vi "parseFloatFromLine.vi"(8 "error in (no error)":errorcluster, 9 "engineeringStatus":string, 10 "line":u32, 11 "DomeCommunicator in":refnum<class "DomeCommunicator.lvclass">) -> (0 "error out":errorcluster, 2 "value":sgl, 3 "DomeCommunicator out":refnum<class "DomeCommunicator.lvclass">)   [LabVIEW 2016, in "DomeCommunicator.lvclass"]
uses:
  DomeCommunicator.lvclass
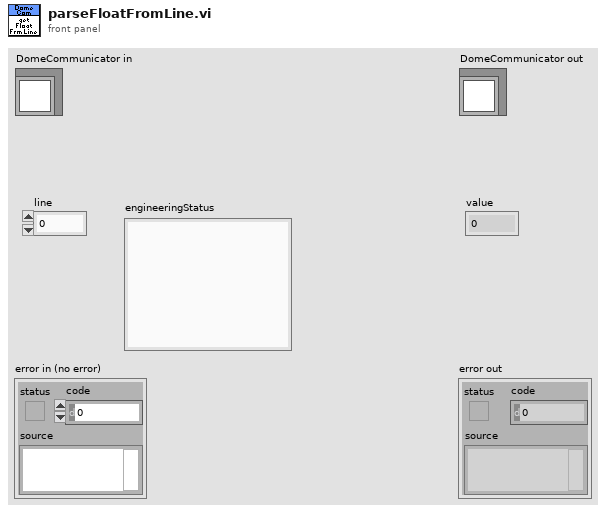
[diagram p1: front panel]
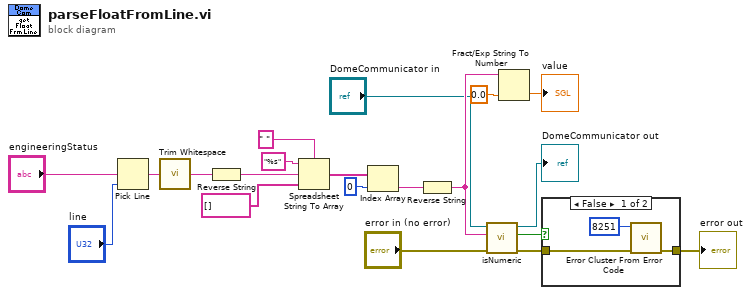
[diagram p0: block diagram]
diagram:
  n1 = Pick Line(multi-line string="engineeringStatus", line index="line") -> (output string=w20:string)  [unwired: 1 in]
  n2 = call <vilib>:"Trim Whitespace.vi"("string"=w20) -> ("trimmed string"=w12:string)  [unwired: 1 in]
  n3 = Reverse String(1:w12) -> (0:w11:string)
  n4 = Spreadsheet String To Array(delimiter (Tab)=" ", format string="%s", spreadsheet string=w11, array type (2D Dbl)=string[] []) -> (array=w15:string[])
  n5 = Index Array(array=w15, index=0) -> (element=w10:string)
  n6 = Reverse String(1:w10) -> (0:w9:string)
  n7 = call "isNumeric.vi"("error in (no error)"="error in (no error)", "numberString"=w9, "DomeCommunicator in"="DomeCommunicator in") -> ("error out"=w13:errorcluster, "isNumeric?"=w14:bool, "DomeCommunicator out"=→"DomeCommunicator out":refnum<class "DomeCommunicator.lvclass">)  [unwired: 6 in]
  n8 = Fract/Exp String To Number(string=w9, default (0 dbl)=sgl 0.0 ("value")) -> (number=→"value":sgl)  [unwired: 2 in, 1 out]
  n9 = case shown="False" w14 {
    tunnel: w13 -> [w22 w24]
    tunnel: [w23 w24] -> w7
    frame False {
      n10 = call <vilib>:"Error Cluster From Error Code.vi"("error in (no error)"=w22, "error code (0)"=8251) -> ("error out"=w23:errorcluster)  [unwired: 7 in]
    }
    frame True {
    }
  }
  "error out" <- w7
